vi "ritter close.vi"(8 "error in (no error)":errorcluster, 11 "VISA in":refnum<visa-resource-name>) -> (0 "error out":errorcluster)   [LabVIEW 2023]
doc: "This vi closes the connection to the gasmeter after clearing the buffers on the serial port."
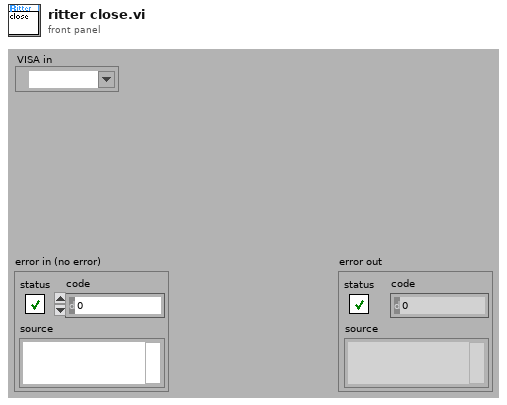
[diagram p1: front panel]
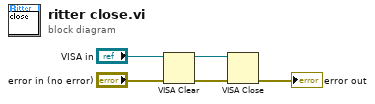
[diagram p0: block diagram]
diagram:
  n1 = VISA Clear(VISA resource name="VISA in", error in (no error)="error in (no error)") -> (VISA resource name out=w5:refnum<visa-resource-name>, error out=w2:errorcluster)
  n2 = VISA Close(VISA resource name=w5, error in (no error)=w2) -> (error out=→"error out":errorcluster)
